vi "FID Rohwerte FGV_F.vi"(0 "Messwerte":u16[](array[numeric]), 5 "Diagnose Werte":u16[](array[numeric]), 7 "Status":bool[](array[boolean]), 9 "Messbereich":u16[](array[numeric]), 13 "Aktion":T1) -> (4 "Messwerte":sgl[](array[numeric]) format="%#.3f", 6 "Diagnose Werte":T3, 8 "Status":T2, 10 "Messbereich":sgl[](array[numeric]) format="%#.3f")   [LabVIEW 2020, in "ABB-EL3000.lvlib" / "FID.lvlib"]
uses:
  FID.lvlib
  Aktion FGV Messwerte_F.ctl
  Allgemeine VI/Allgemeine VI.lvlib
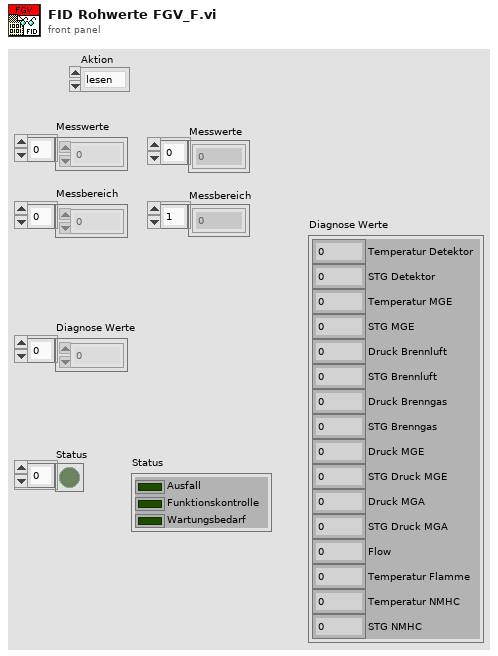
[diagram p1: front panel]
types:
  T1 = typedef "ABB-EL3000.lvlib/FID.lvlib/Aktion FGV Messwerte_F.ctl" = enum16{"lesen", "Messwerte", "Messbereich", "Status", "Diagnose Werte"}
  T2 = cluster{"Ausfall":bool, "Funktionskontrolle":bool, "Wartungsbedarf":bool}
  T3 = cluster{"Temperatur Detektor":sgl, "STG Detektor":sgl, "Temperatur MGE":sgl, "STG MGE":sgl, "Druck Brennluft":sgl, "STG Brennluft":sgl, "Druck Brenngas":sgl, "STG Brenngas":sgl, "Druck MGE":sgl, "STG Druck MGE":sgl, "Druck MGA":sgl, "STG Druck MGA":sgl, "Flow":sgl, "Temperatur Flamme":sgl, "Temperatur NMHC":sgl, "STG NMHC":sgl}
  T4 = cluster{"Status[0]":bool, "Status[1]":bool, "Status[2]":bool}
  T5 = cluster{"Werte[0]":sgl, "Werte[1]":sgl, "Werte[2]":sgl, "Werte[3]":sgl, "Werte[4]":sgl, "Werte[5]":sgl, "Werte[6]":sgl, "Werte[7]":sgl, "Werte[8]":sgl, "Werte[9]":sgl, "Werte[10]":sgl, "Werte[11]":sgl, "Werte[12]":sgl, "Werte[13]":sgl, "Werte[14]":sgl, "Werte[15]":sgl}
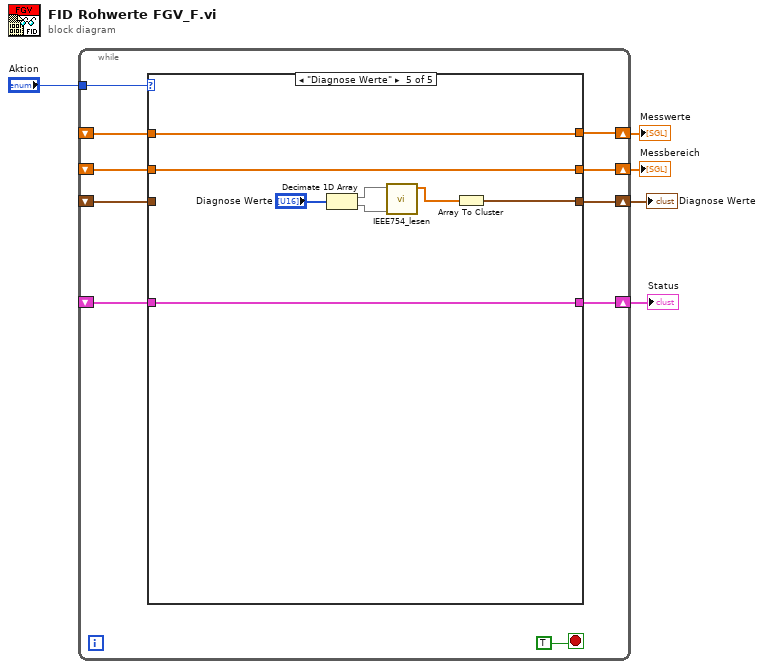
[diagram p0: block diagram]
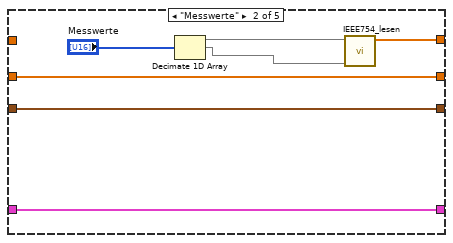
[diagram p3: hidden frame]
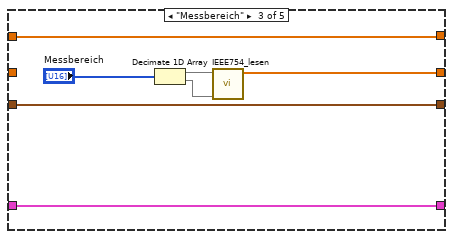
[diagram p4: hidden frame]
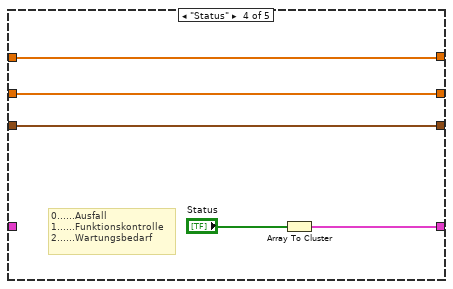
[diagram p5: hidden frame]
diagram:
  n1 = while {
    tunnel: "Aktion" -> [w14]
    shift-right: [w13] -> w5
    shift-left: _ -> [w12]
    shift-right: [w11] -> w4
    shift-left: _ -> [w10]
    shift-right: [w9] -> w3
    shift-left: _ -> [w8]
    shift-right: [w7] -> w2
    shift-left: _ -> [w6]
    stop <- TRUE stop-if-true
    n2 = case shown="\"Diagnose Werte\"" w14 {
      tunnel: [w19 w26 w33 w38 w46] -> w13
      tunnel: w12 -> [w19 _ w33 w38 w46]
      tunnel: [w18 w25 w32 w37 w45] -> w11
      tunnel: w10 -> [w18 w25 _ w37 w45]
      tunnel: [w17 w24 w31 w36 w39] -> w9
      tunnel: w8 -> [w17 w24 w31 w36 _]
      tunnel: [w16 w23 w30 w34 w44] -> w7
      tunnel: w6 -> [w16 w23 w30 _ w44]
      frame "lesen", Default {
      }
      frame "Messwerte" {
        n3 = Decimate 1D Array("Messwerte") -> (w21:u16[], w20:u16[])  [unwired: 1 out]
        n4 = call "IEEE754_lesen.vi"("lo"=w20, "hi"=w21) -> ("Werte"=w26:sgl[])  [unwired: 9 in]
      }
      frame "Messbereich" {
        n5 = Decimate 1D Array("Messbereich") -> (w28:u16[], w27:u16[])
        n6 = call "IEEE754_lesen.vi"("lo"=w27, "hi"=w28) -> ("Werte"=w32:sgl[])  [unwired: 9 in]
      }
      frame "Status" {
        # "0......Ausfall\n1......Funktionskontrolle\n2......Wartungsbedarf"
        n7 = Array To Cluster(array="Status") -> (cluster=w34:T4)
      }
      frame "Diagnose Werte" {
        n8 = Decimate 1D Array("Diagnose Werte") -> (w42:u16[], w41:u16[])
        n9 = call "IEEE754_lesen.vi"("lo"=w41, "hi"=w42) -> ("Werte"=w40:sgl[])  [unwired: 9 in]
        n10 = Array To Cluster(array=w40) -> (cluster=w39:T5)
      }
    }
  }
  "Messwerte" <- w5
  "Messbereich" <- w4
  "Diagnose Werte" <- w3
  "Status" <- w2
